vi "Is Valid.vi"(8 "error in (no error)":errorcluster, 11 "Pub Sub Message Channel in":refnum<class "Pub Sub Message Channel.lvclass">) -> (0 "error out":errorcluster, 2 "Valid":bool, 3 "Pub Sub Message Channel out":refnum<class "Pub Sub Message Channel.lvclass">)   [LabVIEW 2020, in "Actor Pub Sub Channels.lvlib" / "Pub Sub Message Channel.lvclass"]
uses:
  Pub Sub Message Channel.lvclass
  Pub Sub Message Channel.lvclass/Pub Sub Message Channel.ctl
  <vilib>/ActorFramework/Message Queue/Message Queue.lvclass/Message Queue.ctl
  <vilib>/ActorFramework/Message Enqueuer/Message Enqueuer.lvclass
  <vilib>/ActorFramework/Message Dequeuer/Message Dequeuer.lvclass
  <vilib>/ActorFramework/Message Queue/Message Queue.lvclass
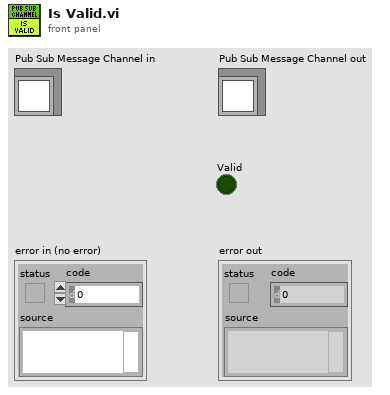
[diagram p1: front panel]
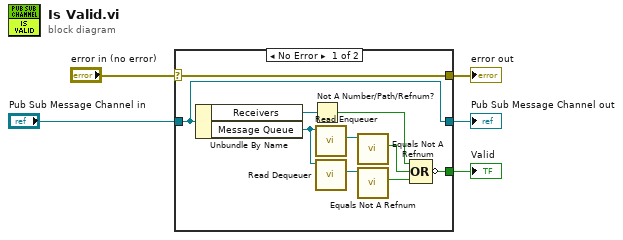
[diagram p0: block diagram]
diagram:
  n1 = case shown="No Error" "error in (no error)" {
    selector: "error in (no error)" -> [w15 w17]
    tunnel: [w15 w17] -> w4
    tunnel: [w14 w16] -> w2
    tunnel: "Pub Sub Message Channel in" -> [w14 w16]
    tunnel: [w6 _] -> w1
    frame No Error {
      n2 = Unbundle By Name(w14) -> ("Receivers"=w13:refnum<data-value>, "Message Queue"=w9:refnum<class "Message Queue.lvclass">)
      n3 = Not A Number/Path/Refnum?(number/path/refnum=w13) -> (NaN/Path/Refnum?=w12:bool)
      n4 = call <vilib>:"Read Enqueuer.vi"("Message Queue"=w9) -> ("Message Enqueuer"=w11:refnum<class "Message Enqueuer.lvclass">)  [unwired: 10 in]
      n5 = call <vilib>:"Read Dequeuer.vi"("Message Queue"=w9) -> ("Message Dequeuer"=w8:refnum<class "Message Dequeuer.lvclass">)  [unwired: 10 in]
      n6 = call <vilib>:"Equals Not A Refnum.vi"("Message Enqueuer"=w11) -> ("Not a refnum?"=w10:bool)  [unwired: 10 in]
      n7 = call <vilib>:"Equals Not A Refnum.vi"("Message Dequeuer"=w8) -> ("Not a refnum?"=w7:bool)  [unwired: 10 in]
      n8 = Compound Arithmetic op=OR(w12, w10, w7) -> (invert w6:bool)
    }
    frame Error {
    }
  }
  "error out" <- w4
  "Pub Sub Message Channel out" <- w2
  "Valid" <- w1
